vi "setLabelVisibility.vi"(8 "error in (no error)":errorcluster, 10 "visibility":bool, 11 "ILabelable in":refnum<class "ILabelable.lvclass">) -> (0 "error out":errorcluster, 3 "ILabelable out":refnum<class "ILabelable.lvclass">)   [LabVIEW 2023, in "TLC_Scripto.lvlib" / "ILabelable.lvclass"]
uses:
  ILabelable.lvclass
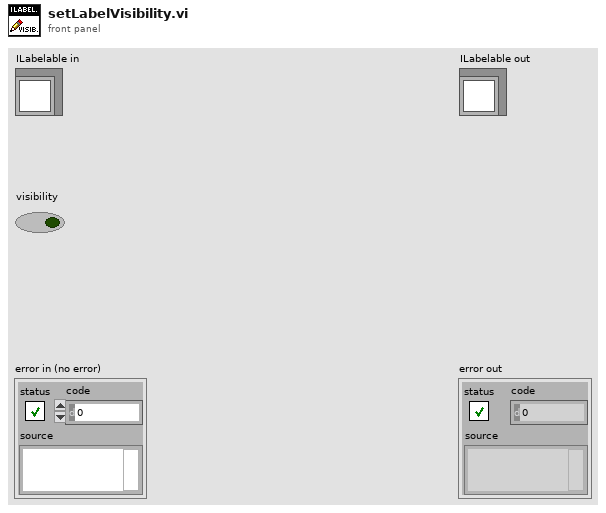
[diagram p1: front panel]
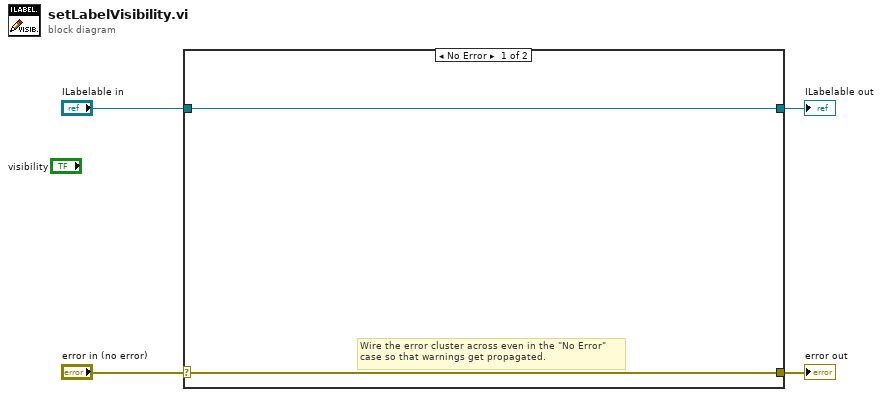
[diagram p0: block diagram]
diagram:
  n1 = case shown="No Error" "error in (no error)" {
    selector: "error in (no error)" -> [w5 w8]
    tunnel: [w5 w8] -> w3
    tunnel: [w6 w7] -> w1
    tunnel: "ILabelable in" -> [w6 w7]
    frame No Error {
      # "Wire the error cluster across even in the \"No Error\"\ncase so that warnings get propagated."
    }
    frame Error {
    }
  }
  "error out" <- w3
  "ILabelable out" <- w1
